vi "RSZVB Channel Add.vi"(8 "error in (no error)":errorcluster {"code" format="%.0x"}, 9 "Channel Name (Ch1)":string="Ch1", 10 "Channel (1)":i32=1, 11 "VISA session":refnum<visa-resource-name>) -> (0 "error out":errorcluster {"code" format="%.0x"}, 3 "dup VISA session":refnum<visa-resource-name>)   [LabVIEW 2011]
doc: "This VI creates channel and selects it as the active channel. It also assigns a name to channel number.\n\nNote(s):\n\nA channel created with CONFigure:CHANnel<Ch>[:STATe] ON can be configured but has no trace assigned so that no measurement can be initiated. Use CALCulate<Ch>:PARameter:SDEFine \"<Trace_name>,\"<Parameter>\" to create a new channel and a new trace.\n\nRemote-control command(s):\nCONFigure:CHANnel<Ch>[:STATe] ON\nCONFigure:CHANnel<Ch>:NAME '<string>'"
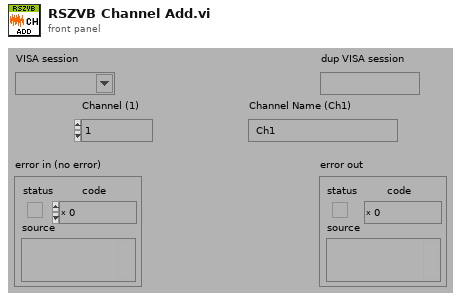
[diagram p1: front panel]
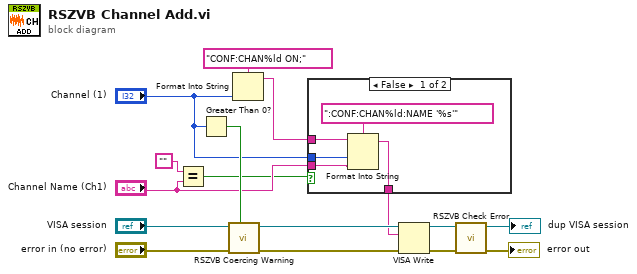
[diagram p0: block diagram]
diagram:
  n1 = Equal?(x="", y="Channel Name (Ch1)") -> (x = y?=w1:bool)
  n2 = Greater Than 0?(x="Channel (1)") -> (x > 0?=w11:bool)
  n3 = call "RSZVB Coercing Warning.vi"("In Range?"=w11, "error in (no error)"="error in (no error)", "VISA session"="VISA session") -> ("error out"=w15:errorcluster, "dup VISA session"=w16:refnum<visa-resource-name>)  [unwired: 7 in]
  n4 = Format Into String(format string="CONF:CHAN%ld ON;", "Channel (1)") -> (resulting string=w4:string)  [unwired: 2 in, 1 out]
  n5 = case shown="False" w1 {
    tunnel: [w20 w22] -> w12
    tunnel: "Channel (1)" -> [w19 _]
    tunnel: w4 -> [w18 w22]
    tunnel: "Channel Name (Ch1)" -> [w17 _]
    frame False {
      n6 = Format Into String(format string=":CONF:CHAN%ld:NAME '%s'", initial string=w18, w19, w17) -> (resulting string=w20:string)  [unwired: 1 in, 1 out]
    }
    frame True {
    }
  }
  n7 = VISA Write(VISA resource name=w16, write buffer=w12, error in (no error)=w15) -> (VISA resource name out=w13:refnum<visa-resource-name>, error out=w14:errorcluster)  [unwired: 1 out]
  n8 = call "RSZVB Check Error.vi"("error in (no error)"=w14, "VISA session"=w13) -> ("error out"=→"error out":errorcluster, "dup VISA session"=→"dup VISA session":refnum<visa-resource-name>)  [unwired: 8 in]
